vi "PID PWM Drive.vi"(8 "PID Gains":cluster{"Kp":dbl, "Kd":dbl, "Ki":dbl}, 9 "Reverse Motor?":bool, 10 "Encoder Position":i32, 11 "Reference":dbl) -> (0 "Control Input":dbl, 2 "Direction":bool, 3 "Duty Cycle":dbl)   [LabVIEW 2018, in "jmslib.lvlib"]
uses:
  jmslib.lvlib
  kevLib2011/Utilities/kCoerceFloat.vi
  kevLib2011.lvlib
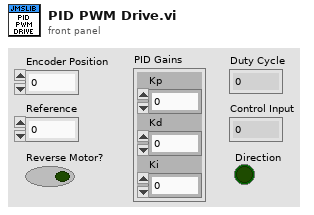
[diagram p1: front panel]
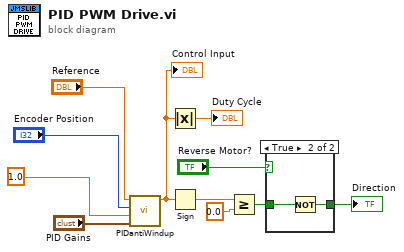
[diagram p0: block diagram]
diagram:
  n1 = call "PIDantiWindup.vi"("PID Gains"="PID Gains", "Saturation"=1.0, "Position"="Encoder Position", "Reference"="Reference") -> ("control"=w11:dbl)  [unwired: 7 in]
  "Control Input" <- w11
  n2 = Absolute Value(x=w11) -> (abs(x)=→"Duty Cycle":dbl)
  n3 = Sign(1:w11) -> (0:w9:dbl)
  n4 = Greater Or Equal?(x=w9, y=0.0) -> (x >= y?=w3:bool)
  n5 = case shown="True" "Reverse Motor?" {
    tunnel: w3 -> [w12 w14]
    tunnel: [w12 w13] -> w2
    frame False {
    }
    frame True {
      n6 = Not(x=w14) -> (.not. x?=w13:bool)
    }
  }
  "Direction" <- w2
